vi "AddControlToWriteVI.vi"(8 "error in (no error)":errorcluster, 11 "BaseAccessorScripter in":refnum<class "BaseAccessorScripter.lvclass">) -> (0 "error out":errorcluster, 3 "BaseAccessorScripter out":refnum<class "BaseAccessorScripter.lvclass">)   [LabVIEW 2021, in "MemberVICreation.lvlib" / "BaseAccessorScripter.lvclass"]
uses:
  <resource>/Framework/Providers/LVClassLibrary/NewAccessors/BaseAccessorScripter/BaseAccessorScripter.lvclass
  <resource>/Framework/Providers/LVClassLibrary/NewAccessors/BaseAccessorScripter/BaseAccessorScripter.lvclass/BaseAccessorScripter.ctl
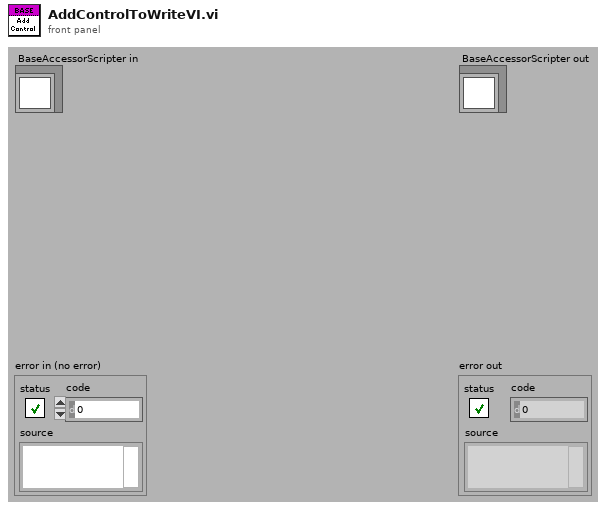
[diagram p1: front panel]
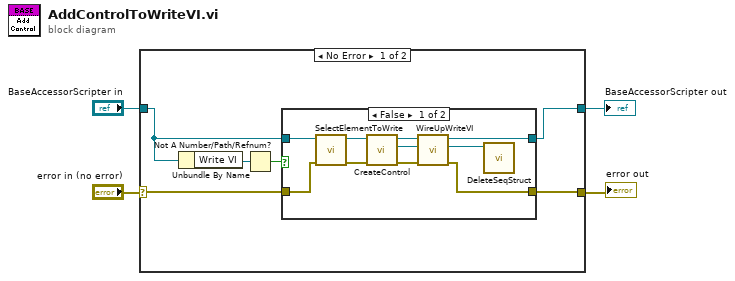
[diagram p0: block diagram]
diagram:
  n1 = case shown="No Error" "error in (no error)" {
    selector: "error in (no error)" -> [w7 w24]
    tunnel: [w6 w24] -> w3
    tunnel: [w5 w23] -> w1
    tunnel: "BaseAccessorScripter in" -> [w8 w23]
    frame No Error {
      n2 = Unbundle By Name(w8) -> ("Write VI"=w10:refnum<vi>)
      n3 = Not A Number/Path/Refnum?(number/path/refnum=w10) -> (NaN/Path/Refnum?=w9:bool)
      n4 = case shown="False" w9 {
        tunnel: w8 -> [w15 w22]
        tunnel: w7 -> [w14 w21]
        tunnel: [w19 w22] -> w5
        tunnel: [w17 w21] -> w6
        frame False {
          n5 = call-dynamic "SelectElementToWrite.vi"("error in (no error)"=w14, "BaseAccessorScripter in"=w15) -> ("error out"=w13:errorcluster, "BaseAccessorScripter out"=w12:refnum<class "BaseAccessorScripter.lvclass">)  [unwired: 8 out]
          n6 = call-dynamic "CreateControl.vi"("error in (no error)"=w13, "BaseAccessorScripter in"=w12) -> ("error out"=w18:errorcluster, "New Control Ref"=w16:refnum<vi>, "BaseAccessorScripter out"=w20:refnum<class "BaseAccessorScripter.lvclass">)  [unwired: 7 out]
          n7 = call-dynamic "WireUpWriteVI.vi"("error in (no error)"=w18, "New Control Ref"=w16, "BaseAccessorScripter in"=w20) -> ("error out"=w17:errorcluster, "Multiframe Stuct out"=w11:refnum<vi>, "BaseAccessorScripter out"=w19:refnum<class "BaseAccessorScripter.lvclass">)  [unwired: 6 out]
          n8 = call <resource>:"DeleteSeqStruct.vi"("Multiframe Stuct in"=w11) -> ()  [unwired: 1 in, 8 out]
        }
        frame True {
        }
      }
    }
    frame Error {
    }
  }
  "error out" <- w3
  "BaseAccessorScripter out" <- w1
